vi "sum_gist1d1.vi"(3 "Y":i16, 5 "hist in":cluster{i16[], i32[]}) -> (1 "hist":cluster{i16[], i32[]})   [LabVIEW 2010]
panel:
  # "Сложение гистограммы с числом"
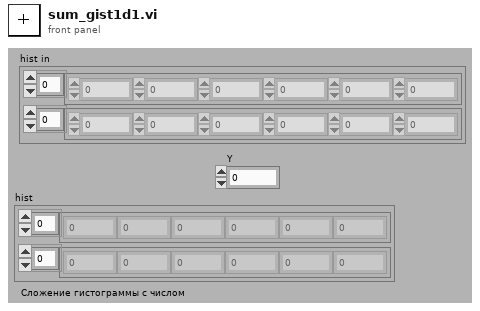
[diagram p1: front panel]
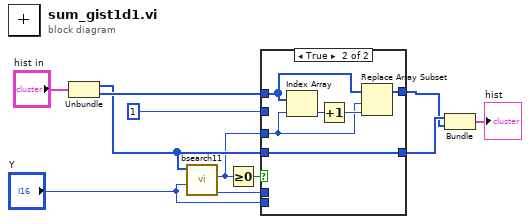
[diagram p0: block diagram]
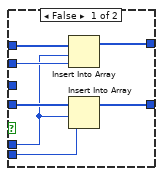
[diagram p2: hidden frame]
diagram:
  n1 = Unbundle("hist in") -> (w4:i16[], w5:i32[])
  n2 = call "bsearch11.vi"("val"="Y", "Array"=w4) -> ("a"=w1:i32, "idx"=w2:i32)  [unwired: 4 in]
  n3 = Greater Or Equal To 0?(x=w2) -> (x >= 0?=w3:bool)
  n4 = case shown="True" w3 {
    tunnel: w4 -> [w18 w24]
    tunnel: [w17 w24] -> w9
    tunnel: "Y" -> [w16 _]
    tunnel: [w15 w20] -> w8
    tunnel: w5 -> [w14 w21]
    tunnel: w2 -> [_ w19]
    tunnel: 1 ("dimension size") -> [w13 _]
    tunnel: w1 -> [w12 _]
    frame False {
      n5 = Insert Into Array(array=w14, index=w12, new element=w13) -> (w15:i32[])
      n6 = Insert Into Array(array=w18, index=w12, new element=w16) -> (w17:i16[])
    }
    frame True {
      n7 = Index Array(array=w21, index=w19) -> (element=w23:i32)
      n8 = Increment(x=w23) -> (x+1=w22:i32)
      n9 = Replace Array Subset(array=w21, new element=w22, index=w19) -> (w20:i32[])
    }
  }
  n10 = Bundle(w9, w8) -> (→"hist":cluster{i16[], i32[]})  [unwired: 1 in]
